vi "MathOperations.vi"(0 "N1":i32, 1 "N6":i32, 2 "N8":i32, 5 "N2":i32, 7 "N3":i32, 9 "N4":i32, 11 "N5":i32, 12 "N7":i32) -> (4 "A":i64, 6 "B":i64)   [LabVIEW 2020]
doc: "This VI takes in 8 numbers in different tabs and perform different math operations on different tabs"
panel:
  in  "?":bool
  in  "Tab Control":enum32{"Page 1", "Page 2", "Page 3", "Page 4"}(tab)
  # "This program performs different math operations in different tabs"
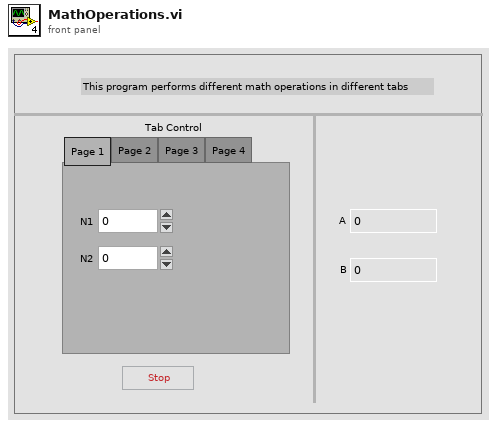
[diagram p1: front panel]
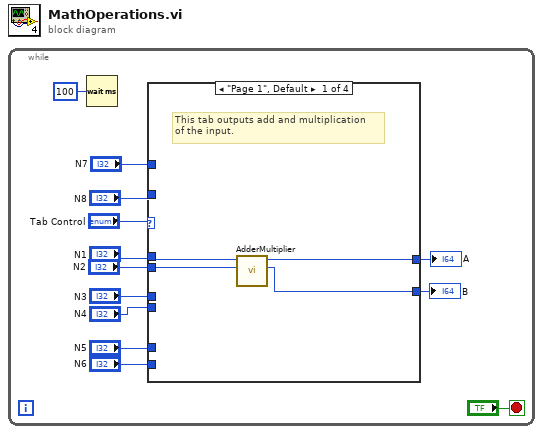
[diagram p0: block diagram]
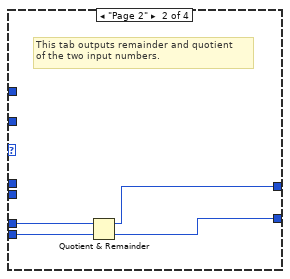
[diagram p2: hidden frame]
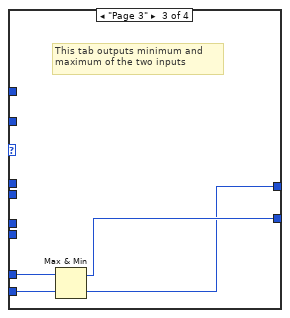
[diagram p3: hidden frame]
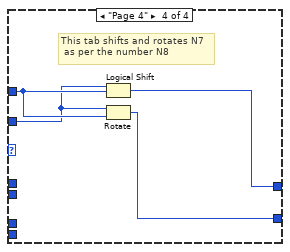
[diagram p4: hidden frame]
diagram:
  n1 = while {
    stop <- "?" stop-if-true
    n2 = Wait (ms)(milliseconds to wait=u32 100) -> ()  [unwired: 1 out]
    n3 = case shown="\"Page 1\", Default" "Tab Control" {
      tunnel: "N1" -> [w17 _ _ _]
      tunnel: "N2" -> [w16 _ _ _]
      tunnel: "N3" -> [_ w21 _ _]
      tunnel: "N4" -> [_ w20 _ _]
      tunnel: "N5" -> [_ _ w25 _]
      tunnel: "N6" -> [_ _ w24 _]
      tunnel: "N7" -> [_ _ _ w29]
      tunnel: "N8" -> [_ _ _ w28]
      tunnel: [w14 w18 w23 w26] -> w4
      tunnel: [w15 w19 w22 w27] -> w3
      frame "Page 1", Default {
        # "This tab outputs add and multiplication\nof the input."
        n4 = call "AdderMultiplier.vi"("N2"=w16, "N1"=w17) -> ("Numeric"=w14:i64, "Numeric 2"=w15:i64)  [unwired: 8 in]
      }
      frame "Page 2" {
        # "This tab outputs remainder and quotient \nof the two input numbers."
        n5 = Quotient & Remainder(x=w21, y=w20) -> (x-y*floor(x/y)=w19:i32, floor(x/y)=w18:i32)
      }
      frame "Page 3" {
        # "This tab outputs minimum and \nmaximum of the two inputs"
        n6 = Max & Min(x=w25, y=w24) -> (max(x,y)=w23:i32, min(x,y)=w22:i32)
      }
      frame "Page 4" {
        # "This tab shifts and rotates N7\n as per the number N8"
        n7 = Logical Shift(y=w28, x=w29) -> (x << y=w27:i32)
        n8 = Rotate(1:w29, 2:w28) -> (0:w26:i32)
      }
    }
    "A" <- w3
    "B" <- w4
  }
